vi "RT_Stepper_Control_Main.vi"() -> ()   [LabVIEW 2019]
uses:
  <vilib>/FPGAPlugInAG/myRIO-1900/niLvFpga_Open_myRIO-1900.vi
  <vilib>/rvi/interface/common/dynamic/niFpgaDynamicAddResources.vi
  <vilib>/Utility/error.llb/Error Cluster From Error Code.vi
  <vilib>/rvi/errors/niLvFpgaAdjustHostInterfaceError.vi
  <vilib>/FPGAPlugInAG/Dynamic/niLvFpga_Close_Dynamic.vi
  <vilib>/rvi/interface/nirviOpenFPGA/nirviOpenFPGA.xnode
  FPGA Bitfiles/StepperControl_FPGATarget_FPGAStepperContr_5sjZJBEegh8.lvbitx
  FPGA_Stepper_Control_Main.vi
  <vilib>/rvi/interface/nirviReadWriteControl/nirviReadWriteControl.xnode
  <vilib>/rvi/interface/nirviCloseFPGA/nirviCloseFPGA.xnode
  NiFpgaLv.dll
  <vilib>/rvi/interface/Simulation/niFpgaSimulationCallBeginRW.vi
panel:
  in  "stop":bool
  in  "Stepper Direction":bool
  in  "Stepper Enable":bool
  in  "Half Peirod (pulse 40MHz)":u32
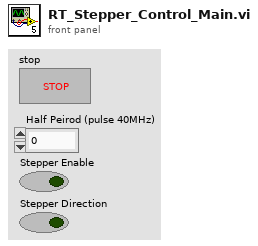
[diagram p1: front panel]
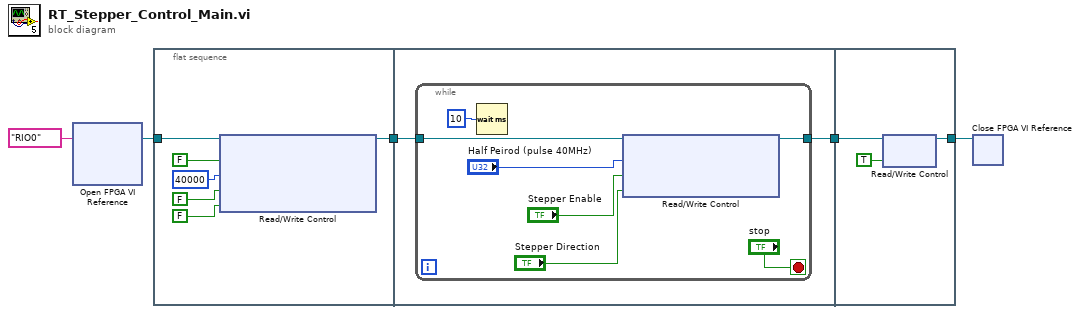
[diagram p0: block diagram]
diagram:
  n1 = xnode "Open FPGA VI Reference"("resource name"=tag "RIO0") -> ("FPGA VI Reference Out"=w4:refnum<k20>)  [unwired: 1 in, 1 out]
  n2 = flat-sequence {
    tunnel: w4 -> [w11]
    tunnel: [w10] -> w3
    tunnel: w3 -> [w13]
    tunnel: [w12] -> w2
    tunnel: w2 -> [w23]
    tunnel: [w22] -> w1
    frame #0 {
      n3 = xnode "Read/Write Control"("FPGA VI Reference In"=w11, "stop"=FALSE, "Half Peirod (pulse 40MHz)"=u32 40000, "Stepper Enable"=FALSE, "Stepper Direction"=FALSE) -> ("FPGA VI Reference Out"=w10:refnum<k20>)  [unwired: 1 in, 1 out]
    }
    frame #1 {
      n4 = while {
        tunnel: w13 -> [w20]
        tunnel: [w19] -> w12
        stop <- "stop" stop-if-true
        n5 = Wait (ms)(milliseconds to wait=u32 10) -> ()  [unwired: 1 out]
        n6 = xnode "Read/Write Control"("FPGA VI Reference In"=w20, "Half Peirod (pulse 40MHz)"="Half Peirod (pulse 40MHz)", "Stepper Enable"="Stepper Enable", "Stepper Direction"="Stepper Direction") -> ("FPGA VI Reference Out"=w19:refnum<k20>)  [unwired: 1 in, 1 out]
      }
    }
    frame #2 {
      n7 = xnode "Read/Write Control"("FPGA VI Reference In"=w23, "stop"=TRUE) -> ("FPGA VI Reference Out"=w22:refnum<k20>)  [unwired: 1 in, 1 out]
    }
  }
  n8 = xnode "Close FPGA VI Reference"("FPGA VI Reference In"=w1) -> ()  [unwired: 1 in, 1 out]
